vi "Update Templates Pluck EncodedParameters for Spartan 5.0.vi"(8 "error in (no error)":errorcluster, 11 "Connection Refnum":T1) -> (0 "error out":errorcluster, 2 "EncodedParameters":string[](array[string]), 3 "Connection Refnum":T1)   [LabVIEW 2011]
uses:
  SI.LIB/ODBC/SQL Controls/Connection Refnum.ctl
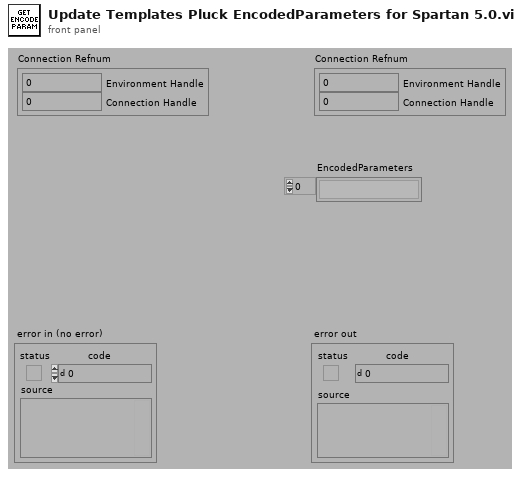
[diagram p1: front panel]
types:
  T1 = typedef "Connection Refnum.ctl" = cluster{"Environment Handle":i32, "Connection Handle":i32}
  T2 = typedef "Statement Refnum.ctl" = cluster{"Statement Handle":i32, "Parameter Number":u16}
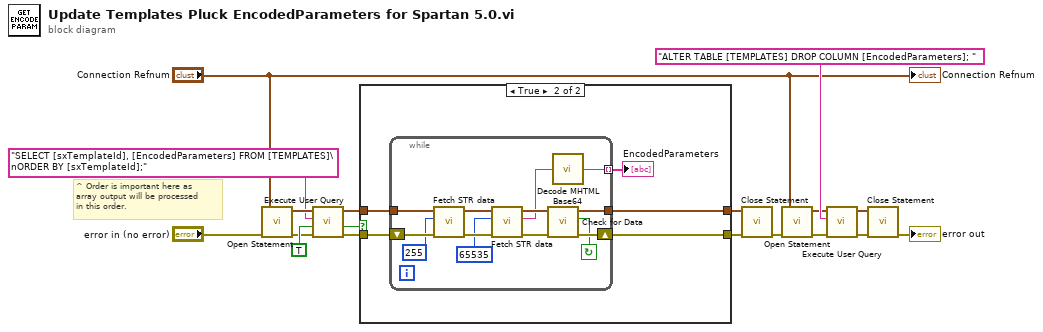
[diagram p0: block diagram]
diagram:
  # "^ Order is important here as\narray output will be processed\nin this order."
  n1 = call "Open Statement.vi"("error in (no error)"="error in (no error)", "Connection Refnum"="Connection Refnum") -> ("error out"=w17:errorcluster, "Statement Refnum"=w15:T2)  [unwired: 4 out]
  n2 = call "Execute User Query.vi"("error in (no error)"=w17, "Return Data? (f)"=TRUE, "User Query"="SELECT [sxTemplateId], [EncodedParameters] FROM [TEMPLATES]\nORDER BY [sxTemplateId];", "Statement Refnum"=w15) -> ("error out"=w11:errorcluster, "Data Present?"=w12:bool, "Statement Refnum"=w13:T2)  [unwired: 1 out]
  n3 = case shown="True" w12 {
    tunnel: w13 -> [w19 w24]
    tunnel: w11 -> [w20 w25]
    tunnel: [w20 w23] -> w8
    tunnel: [w19 w22] -> w9
    frame False {
    }
    frame True {
      n4 = while {
        shift-right: [w38] -> w23
        shift-left: w25 -> [w31]
        tunnel: w24 -> [w33]
        tunnel: [w37] -> w22
        tunnel: [w26] -> w21 mode=indexing
        stop <- w36 continue-if-true
        n5 = call "Fetch STR data.vi"("error in (no error)"=w31, "Buffer Size"=255, "Statement Refnum"=w33) -> ("error out"=w30:errorcluster, "Statement Refnum"=w32:T2)  [unwired: 3 out]
        n6 = call "Fetch STR data.vi"("error in (no error)"=w30, "Buffer Size"=65535, "Statement Refnum"=w32) -> ("error out"=w34:errorcluster, "Data"=w27:string, "Statement Refnum"=w35:T2)  [unwired: 2 out]
        n7 = call "Check for Data.vi"("error in (no error)"=w34, "Statement Refnum"=w35) -> ("error out"=w38:errorcluster, "Data Present?"=w36:bool, "Statement Refnum"=w37:T2)  [unwired: 3 out]
        n8 = call "Decode MHTML Base64.vi"("Encoded String\n(Base64)"=w27) -> ("Decoded Binary\nString"=w26:string)  [unwired: 14 out]
      }
      "EncodedParameters" <- w21
    }
  }
  n9 = call "Close Statement.vi"("error in (no error)"=w8, "Statement Refnum"=w9) -> ("error out"=w2:errorcluster)  [unwired: 5 out]
  n10 = call "Open Statement.vi"("error in (no error)"=w2, "Connection Refnum"="Connection Refnum") -> ("error out"=w4:errorcluster, "Statement Refnum"=w3:T2)  [unwired: 4 out]
  n11 = call "Execute User Query.vi"("error in (no error)"=w4, "User Query"="ALTER TABLE [TEMPLATES] DROP COLUMN [EncodedParameters]; ", "Statement Refnum"=w3) -> ("error out"=w6:errorcluster, "Statement Refnum"=w7:T2)  [unwired: 1 in, 2 out]
  n12 = call "Close Statement.vi"("error in (no error)"=w6, "Statement Refnum"=w7) -> ("error out"=→"error out":errorcluster)  [unwired: 5 out]
  "Connection Refnum" <- "Connection Refnum"
